vi "Write states.vi"(8 "error in (no error)":errorcluster, 10 "States":T1, 11 "SupportAttackerRole in":refnum<class "SupportAttackerRole.lvclass">) -> (0 "error out":errorcluster, 3 "SupportAttackerRole out":refnum<class "SupportAttackerRole.lvclass">)   [LabVIEW 2023, in "SupportAttackerRole.lvclass"]
uses:
  SupportAttackerRole.lvclass
  SupportAttackerRole_states.ctl
  SupportAttackerRole.lvclass/SupportAttackerRole.ctl
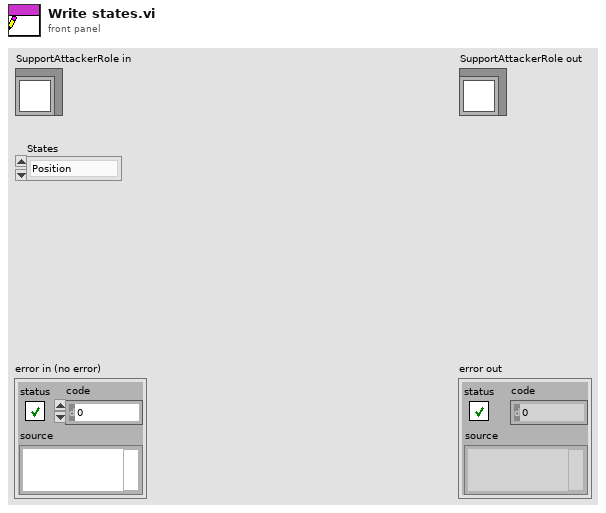
[diagram p1: front panel]
types:
  T1 = typedef "SupportAttackerRole.lvclass/SupportAttackerRole_states.ctl" = enum16{"Position", "WaitPass", "Exit"}
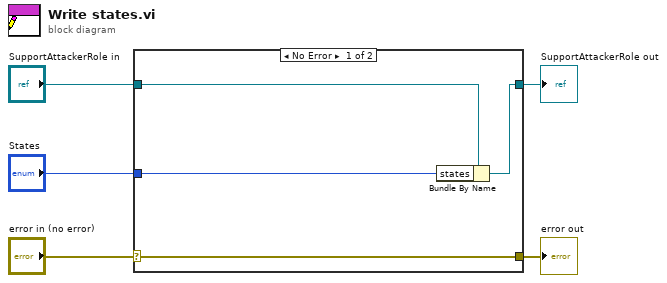
[diagram p0: block diagram]
diagram:
  n1 = case shown="No Error" "error in (no error)" {
    selector: "error in (no error)" -> [w9 w10]
    tunnel: [w9 w10] -> w4
    tunnel: [w7 w11] -> w2
    tunnel: "SupportAttackerRole in" -> [w8 w11]
    tunnel: "States" -> [w6 _]
    frame No Error {
      n2 = Bundle By Name(cluster=w8, "states"=w6) -> (w7:refnum<class "SupportAttackerRole.lvclass">)
    }
    frame Error {
    }
  }
  "error out" <- w4
  "SupportAttackerRole out" <- w2
